vi "FTW-CodeGen-Prototype.vi"(0 "REPLACED_SQLite Connector":refnum<class "FTW-SQLite-Connector.lvclass">, 2 "REPLACED_SQL Script":string, 5 "ADAPT_Row Datatype":cluster{"Column":variant}, 11 "REPLACED_error in":errorcluster) -> (4 "REPLACED_SQLite Connector out":refnum<class "FTW-SQLite-Connector.lvclass">, 6 "ADAPT_Result Set":cluster{"Column":variant}[](array[cluster]), 8 "REPLACED_Time to Execute+Compile":dbl format="%.6fsec", 10 "REPLACED_Time to Compile SQL":dbl format="%.6fsec", 15 "REPLACED_error out":errorcluster)   [LabVIEW 2013, in "FTW-SQLite-Fetch.xnode"]
uses:
  FTW-SQLite-Fetch.xnode
  src/Database/FTW-SQLite-Connector.lvclass
panel:
  # "Inputs"
  # "Outputs"
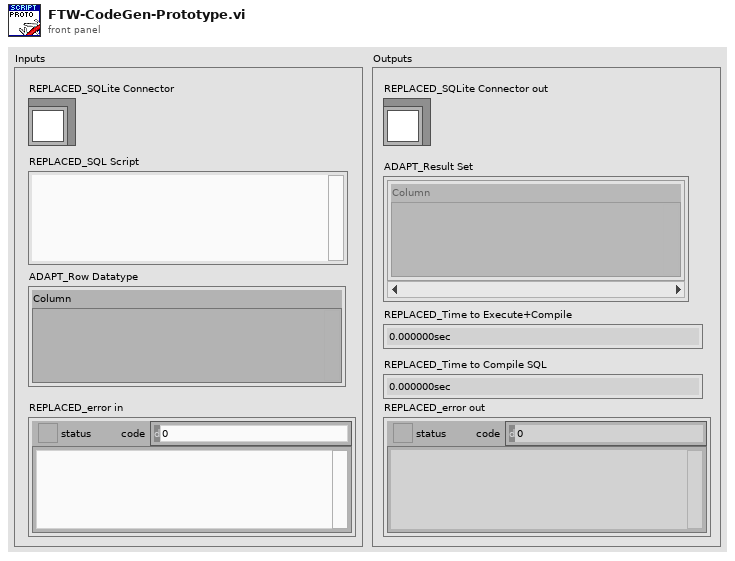
[diagram p1: front panel]
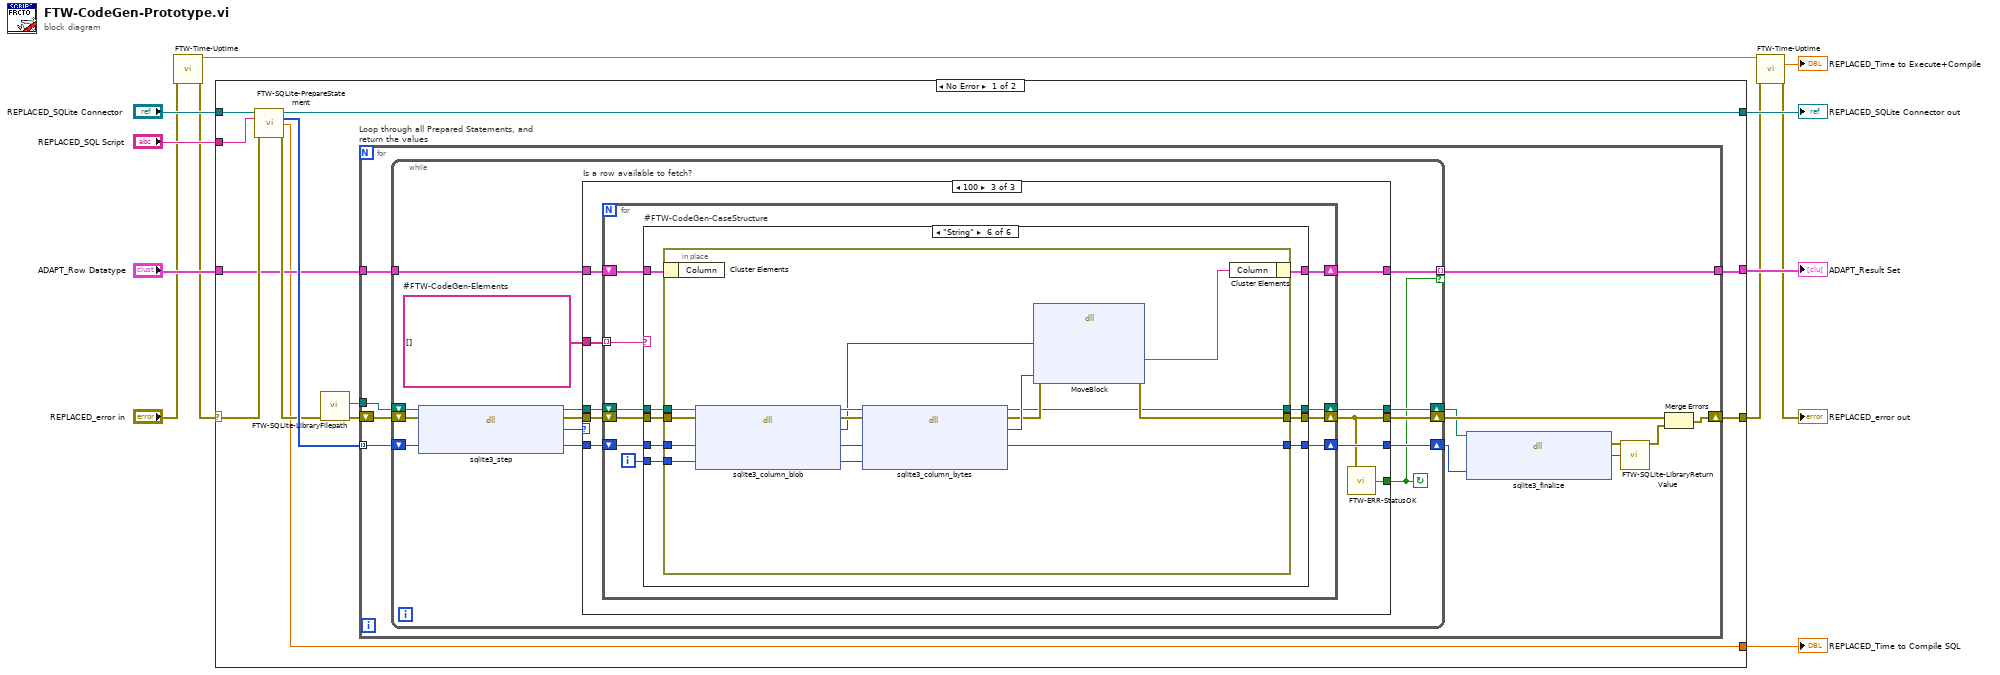
[diagram p0: block diagram]
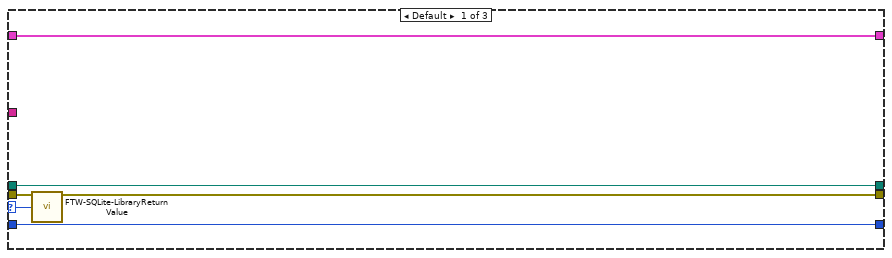
[diagram p2: hidden frame]
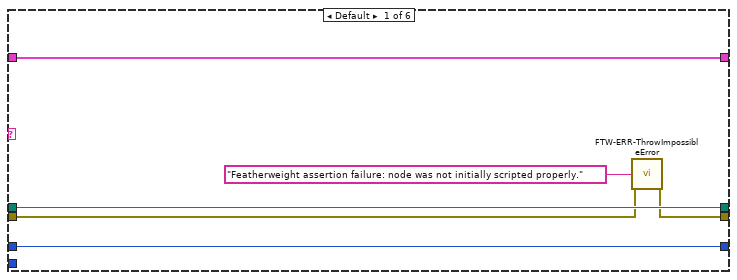
[diagram p4: hidden frame]
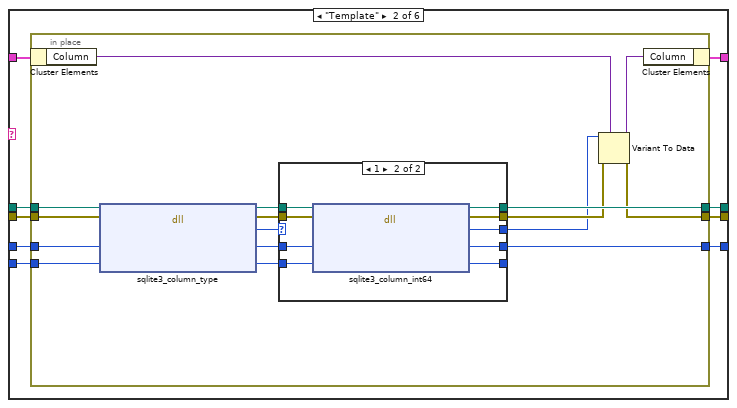
[diagram p5: hidden frame]
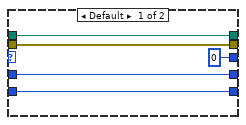
[diagram p6: hidden frame]
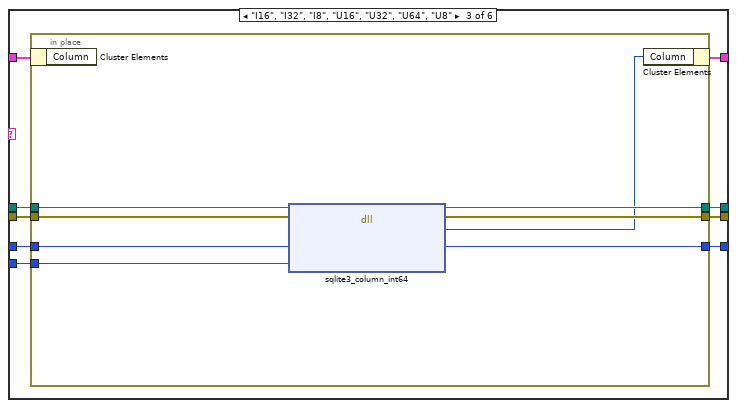
[diagram p7: hidden frame]
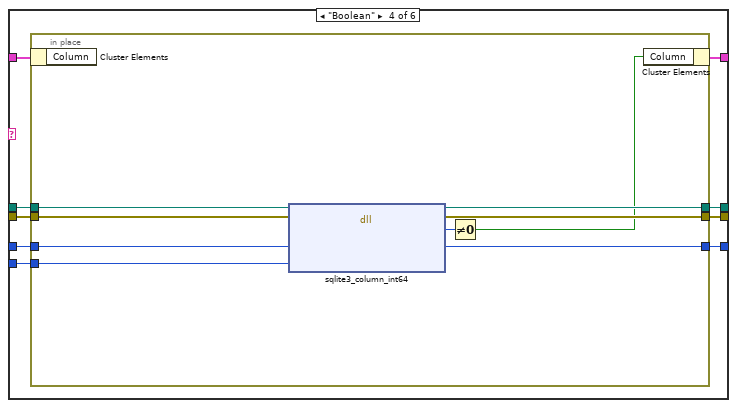
[diagram p8: hidden frame]
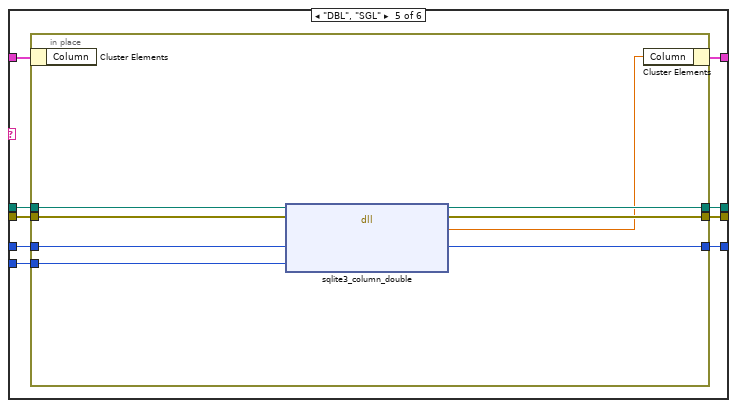
[diagram p9: hidden frame]
diagram:
  n1 = call "FTW-Time-Uptime.vi"("error in"="REPLACED_error in") -> ("Current Uptime"=w3:dbl, "error out"=w6:errorcluster)  [unwired: 12 in, 1 out]
  n2 = case shown="No Error" w6 {
    selector: w6 -> [w23 w202]
    tunnel: "REPLACED_SQLite Connector" -> [w24 w203]
    tunnel: [w22 w203] -> w11
    tunnel: "REPLACED_SQL Script" -> [w21 _]
    tunnel: [w16 w202] -> w4
    tunnel: "ADAPT_Row Datatype" -> [w14 _]
    tunnel: [w15 _] -> w8
    tunnel: [w13 _] -> w1
    frame No Error {
      n3 = call "FTW-SQLite-PrepareStatement.vi"("SQLite Connector"=w24, "SQL Statement"=w21, "error in"=w23) -> ("SQLite Connector out"=w22:refnum<class "FTW-SQLite-Connector.lvclass">, "Prepared Statements"=w20:i64[], "Time to Compile SQL"=w13:dbl, "error out"=w19:errorcluster)  [unwired: 9 in]
      n4 = call "FTW-SQLite-LibraryFilepath.vi"("error in"=w19) -> ("error out"=w18:errorcluster, "SQLite Library Filepath"=w17:path)  [unwired: 8 in, 1 out]
      n5 = for "Loop through all Prepared Statements, and return the values" {
        tunnel: w20 -> [w26] mode=indexing
        shift-right: [w34] -> w16
        shift-left: w18 -> [w27]
        tunnel: w17 -> [w28]
        tunnel: w14 -> [w29]
        tunnel: [w25] -> w15
        n6 = while {
          shift-right: [w41] -> w30
          shift-left: w28 -> [w49]
          shift-right: [w43] -> w32
          shift-left: w27 -> [w50]
          shift-right: [w42] -> w31
          shift-left: w26 -> [w48]
          tunnel: w29 -> [w38]
          tunnel: [w40] -> w25 mode=indexing if=w39
          stop <- w39 continue-if-true
          w37 = string[] []  # #FTW-CodeGen-Elements
          n7 = dll-call lib="?" fn="sqlite3_step"(path in=w49, error in=w50, "Prepared Statement Pointer"=w48) -> (path out=w44:path, error out=w46:errorcluster, "Return Value"=w47:i32, "Prepared Statement Pointer"=w45:i64)  [unwired: 1 in]
          n8 = case "Is a row available to fetch?" shown="100" w47 {
            selector: w47 -> [w56 _ _]
            tunnel: w46 -> [w55 w60 w69]
            tunnel: w45 -> [w53 w58 w68]
            tunnel: w44 -> [w52 w59 w70]
            tunnel: [w54 w60 w64] -> w43
            tunnel: [w53 w58 w66] -> w42
            tunnel: [w52 w59 w67] -> w41
            tunnel: w38 -> [w51 w57 w63]
            tunnel: [_ _ w65] -> w39
            tunnel: [w51 w57 w62] -> w40
            tunnel: w37 -> [_ _ w61]
            frame Default {
              n9 = call "FTW-SQLite-LibraryReturnValue.vi"("error in"=w55, "Return Value"=w56) -> ("error out"=w54:errorcluster)  [unwired: 13 in]
            }
            frame 101 {
              # "SQLITE_DONE=101 -- looks like there are no more columns to fetch!"
            }
            frame 100 {
              n10 = for {
                shift-right: [w77] -> w67
                shift-left: w70 -> [w80]
                shift-right: [w75] -> w64
                shift-left: w69 -> [w79]
                shift-right: [w76] -> w66
                shift-left: w68 -> [w78]
                shift-right: [w73] -> w62
                shift-left: w63 -> [w74]
                tunnel: w61 -> [w71] mode=indexing
                i -> [w72]
                n11 = case "#FTW-CodeGen-CaseStructure" shown="\"String\"" w71 {
                  tunnel: w80 -> [w86 w95 w131 w148 w166 w185]
                  tunnel: w79 -> [w83 w94 w130 w147 w165 w184]
                  tunnel: w78 -> [w85 w93 w129 w146 w164 w183]
                  tunnel: [w86 w92 w134 w151 w169 w181] -> w77
                  tunnel: [w85 w91 w133 w150 w168 w180] -> w76
                  tunnel: [w82 w90 w132 w149 w167 w186] -> w75
                  tunnel: w74 -> [w84 w89 w127 w144 w162 w179]
                  tunnel: [w84 w88 w126 w143 w161 w178] -> w73
                  tunnel: w72 -> [_ w87 w128 w145 w163 w182]
                  frame Default {
                    n12 = call "FTW-ERR-ThrowImpossibleError.vi"("Reason this error should never happen"="Featherweight assertion failure: node was not initially scripted properly.", "error in"=w83) -> ("error out"=w82:errorcluster)  [unwired: 13 in]
                  }
                  frame "Template" {
                    n13 = in-place "In Place Element Structure" {
                      in-place-border: w95 -> [w111]
                      in-place-border: w94 -> [w110]
                      in-place-border: w93 -> [w109]
                      in-place-border: [w108] -> w92
                      in-place-border: [w107] -> w91
                      in-place-border: [w100] -> w90
                      in-place-border: w87 -> [w101]
                      n14 = in-place-cluster #1 ("Unbundle / Bundle Elements")(w89) -> ("Column"=w98:variant)
                      n15 = dll-call lib="?" fn="sqlite3_column_type"(path in=w111, error in=w110, "Prepared Statement Pointer"=w109, "Column Index"=w101) -> (path out=w103:path, error out=w102:errorcluster, "Column Type"=w106:i32, "Prepared Statement Pointer"=w104:i64, "Column Index"=w105:i32)  [unwired: 1 in]
                      n16 = case shown="1" w106 {
                        tunnel: w105 -> [w113 w124]
                        tunnel: w104 -> [w114 w125]
                        tunnel: w103 -> [w116 w123]
                        tunnel: w102 -> [w115 w122]
                        tunnel: [w116 w121] -> w108
                        tunnel: [w115 w120] -> w99
                        tunnel: [w114 w119] -> w107
                        tunnel: [w113 w118] -> _
                        tunnel: [i64 0 ("I64 Value") w117] -> w96
                        frame Default {
                        }
                        frame 1 {
                          n17 = dll-call lib="?" fn="sqlite3_column_int64"(path in=w123, error in=w122, "Prepared Statement Pointer"=w125, "Column Index"=w124) -> (path out=w121:path, error out=w120:errorcluster, "I64 Value"=w117:i64, "Prepared Statement Pointer"=w119:i64, "Column Index"=w118:i32)  [unwired: 1 in]
                        }
                      }
                      n18 = Variant To Data(error in=w99, type=w98, Variant=w96) -> (data=w97:variant, error out=w100:errorcluster)
                      n19 = in-place-cluster #1 ("Unbundle / Bundle Elements")("Column"=w97) -> (w88:cluster{"Column":variant})
                    }
                  }
                  frame "I16", "I32", "I8", "U16", "U32", "U64", "U8" {
                    n20 = in-place "In Place Element Structure" {
                      in-place-border: [w142] -> w134
                      in-place-border: [w141] -> w133
                      in-place-border: [w140] -> w132
                      in-place-border: w131 -> [w139]
                      in-place-border: w130 -> [w138]
                      in-place-border: w129 -> [w137]
                      in-place-border: w128 -> [w136]
                      n21 = in-place-cluster #2 ("Unbundle / Bundle Elements")(w127) -> ()  [unwired: 1 out]
                      n22 = dll-call lib="?" fn="sqlite3_column_int64"(path in=w139, error in=w138, "Prepared Statement Pointer"=w137, "Column Index"=w136) -> (path out=w142:path, error out=w140:errorcluster, "I64 Value"=w135:i64, "Prepared Statement Pointer"=w141:i64)  [unwired: 2 in]
                      n23 = in-place-cluster #2 ("Unbundle / Bundle Elements")("Column"=w135) -> (w126:cluster{"Column":variant})
                    }
                  }
                  frame "Boolean" {
                    n24 = in-place "In Place Element Structure" {
                      in-place-border: [w160] -> w151
                      in-place-border: [w159] -> w150
                      in-place-border: [w158] -> w149
                      in-place-border: w148 -> [w157]
                      in-place-border: w147 -> [w156]
                      in-place-border: w146 -> [w155]
                      in-place-border: w145 -> [w154]
                      n25 = in-place-cluster #3 ("Unbundle / Bundle Elements")(w144) -> ()  [unwired: 1 out]
                      n26 = dll-call lib="?" fn="sqlite3_column_int64"(path in=w157, error in=w156, "Prepared Statement Pointer"=w155, "Column Index"=w154) -> (path out=w160:path, error out=w158:errorcluster, "I64 Value"=w153:i64, "Prepared Statement Pointer"=w159:i64)  [unwired: 2 in]
                      n27 = Not Equal To 0?(x=w153) -> (x != 0?=w152:bool)
                      n28 = in-place-cluster #3 ("Unbundle / Bundle Elements")("Column"=w152) -> (w143:cluster{"Column":variant})
                    }
                  }
                  frame "DBL", "SGL" {
                    n29 = in-place "In Place Element Structure" {
                      in-place-border: [w177] -> w169
                      in-place-border: [w176] -> w168
                      in-place-border: [w175] -> w167
                      in-place-border: w166 -> [w174]
                      in-place-border: w165 -> [w173]
                      in-place-border: w164 -> [w172]
                      in-place-border: w163 -> [w171]
                      n30 = in-place-cluster #4 ("Unbundle / Bundle Elements")(w162) -> ()  [unwired: 1 out]
                      n31 = dll-call lib="?" fn="sqlite3_column_double"(path in=w174, error in=w173, "Prepared Statement Pointer"=w172, "Column Index"=w171) -> (path out=w177:path, error out=w175:errorcluster, "DBL Value"=w170:dbl, "Prepared Statement Pointer"=w176:i64)  [unwired: 2 in]
                      n32 = in-place-cluster #4 ("Unbundle / Bundle Elements")("Column"=w170) -> (w161:cluster{"Column":variant})
                    }
                  }
                  frame "String" {
                    n33 = in-place "In Place Element Structure" {
                      in-place-border: [w201] -> w186
                      in-place-border: w185 -> [w199]
                      in-place-border: w184 -> [w198]
                      in-place-border: w183 -> [w197]
                      in-place-border: w182 -> [w196]
                      in-place-border: [w189] -> w181
                      in-place-border: [w188] -> w180
                      n34 = in-place-cluster #5 ("Unbundle / Bundle Elements")(w179) -> ()  [unwired: 1 out]
                      n35 = dll-call lib="?" fn="sqlite3_column_blob"(path in=w199, error in=w198, "Prepared Statement Pointer"=w197, "Column Index"=w196) -> (path out=w195:path, error out=w194:errorcluster, "BLOB Pointer"=w191:i64, "Prepared Statement Pointer"=w193:i64, "Column Index"=w192:i32)  [unwired: 1 in]
                      n36 = dll-call lib="?" fn="sqlite3_column_bytes"(path in=w195, error in=w194, "Prepared Statement Pointer"=w193, "Column Index"=w192) -> (path out=w189:path, error out=w190:errorcluster, "BLOB Size"=w200:i32, "Prepared Statement Pointer"=w188:i64)  [unwired: 2 in]
                      n37 = dll-call lib="LabVIEW" fn="MoveBlock"(error in=w190, "BLOB Source Pointer"=w191, "BLOB Size"=w200) -> (error out=w201:errorcluster, "BLOB Destination"=w187:string)  [unwired: 6 in, 1 out]
                      n38 = in-place-cluster #5 ("Unbundle / Bundle Elements")("Column"=w187) -> (w178:cluster{"Column":variant})
                    }
                  }
                }
              }
              n39 = call "FTW-ERR-StatusOK.vi"("error to check"=w64) -> ("Status OK?"=w65:bool)
            }
          }
        }
        n40 = dll-call lib="?" fn="sqlite3_finalize"(path in=w30, "Prepared Statement Pointer"=w31) -> (error out=w36:errorcluster, "Return Value"=w35:i32)  [unwired: 3 in, 1 out]
        n41 = call "FTW-SQLite-LibraryReturnValue.vi"("error in"=w36, "Return Value"=w35) -> ("error out"=w33:errorcluster)  [unwired: 13 in]
        n42 = Merge Errors(w32, w33) -> (w34:errorcluster)
      }
    }
    frame Error {
    }
  }
  "REPLACED_SQLite Connector out" <- w11
  "ADAPT_Result Set" <- w8
  "REPLACED_Time to Compile SQL" <- w1
  n43 = call "FTW-Time-Uptime.vi"("Previous Uptime"=w3, "error in"=w4) -> ("Elapsed Time"=→"REPLACED_Time to Execute+Compile":dbl, "error out"=→"REPLACED_error out":errorcluster)  [unwired: 11 in, 1 out]
